vi "CMD_SERIALPARSE.vi"(6 "Gantry in":refnum<class "Gantry.lvclass">, 7 "Console Log in":refnum<class "Console Log.lvclass">, 8 "error in (no error)":errorcluster, 10 "Arguments":string[](array[string]), 11 "gScript Interpreter in":refnum<class "gScript Interpreter.lvclass">) -> (0 "error out":errorcluster, 3 "gScript Interpreter out":refnum<class "gScript Interpreter.lvclass">, 4 "Gantry out":refnum<class "Gantry.lvclass">, 5 "Console Log out":refnum<class "Console Log.lvclass">)   [LabVIEW 2024, in "gScript Interpreter.lvclass"]
uses:
  gScript Interpreter.lvclass
  Shared Components/Gantry Class/Gantry.lvclass
  Application Utilities/Console Log/Console Log.lvclass
  Type Definitions/Memory Cell.ctl
  Type Definitions/Memory Cell Type Enum.ctl
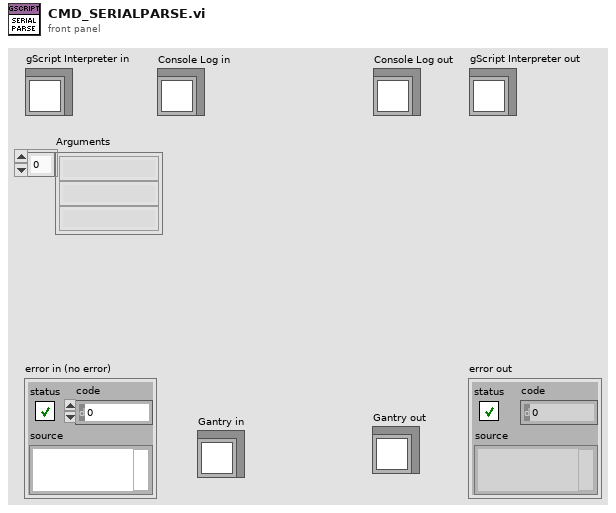
[diagram p1: front panel]
types:
  T1 = typedef "Memory Cell.ctl" = cluster{"type":T2, "x":dbl, "y":dbl, "z":dbl, "w":dbl}
  T2 = typedef "Memory Cell Type Enum.ctl" = enum16{"integer", "float", "vector", "rotation"}
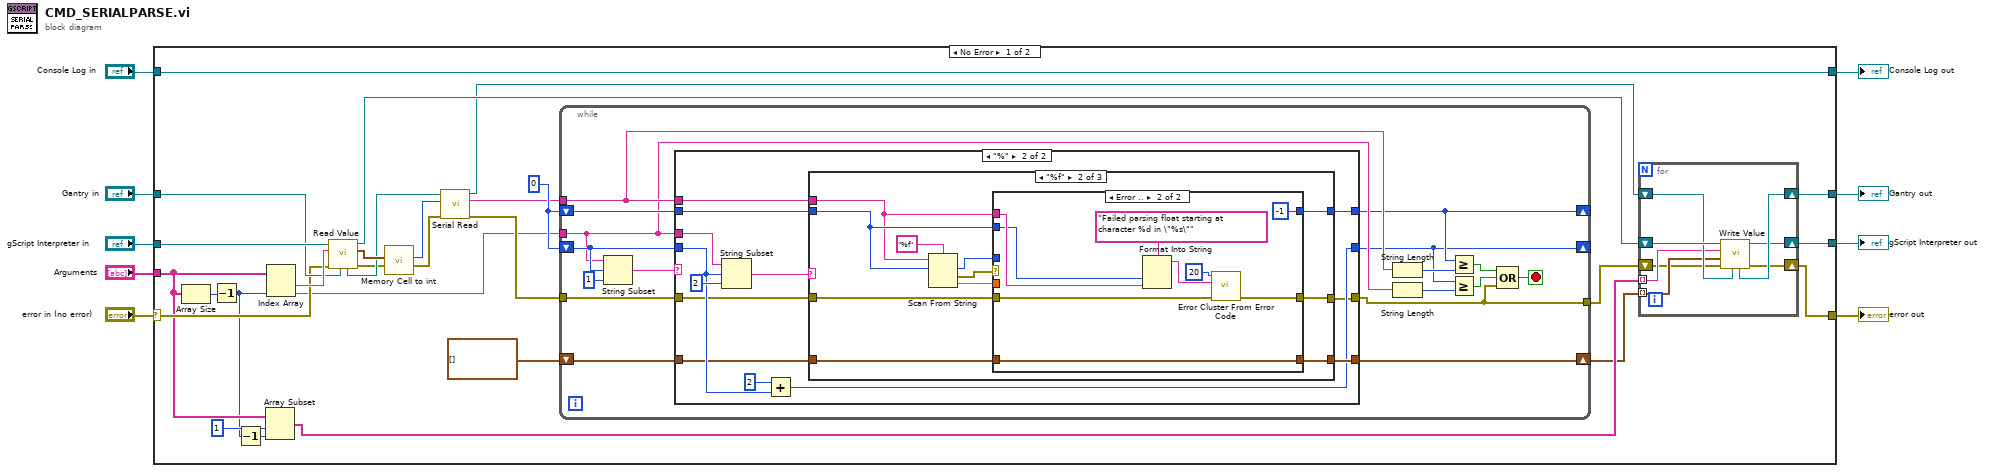
[diagram p0: block diagram]
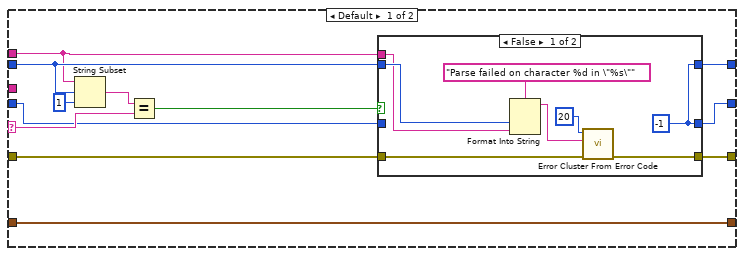
[diagram p2: hidden frame]
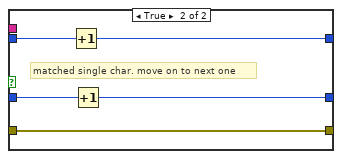
[diagram p3: hidden frame]
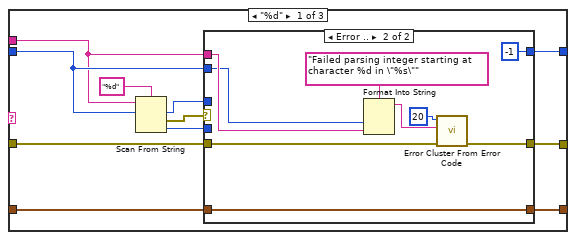
[diagram p4: hidden frame]
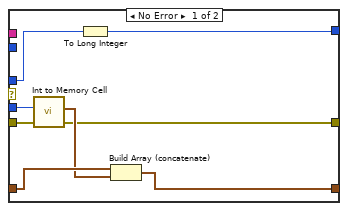
[diagram p5: hidden frame]
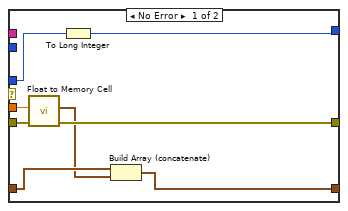
[diagram p6: hidden frame]
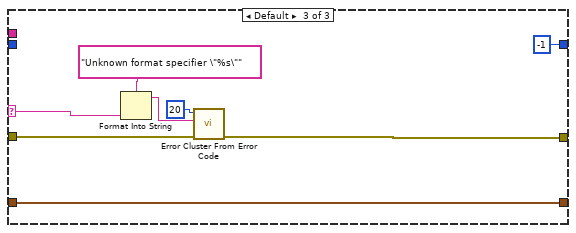
[diagram p7: hidden frame]
diagram:
  n1 = case shown="No Error" "error in (no error)" {
    selector: "error in (no error)" -> [w32 w165]
    tunnel: [w10 w165] -> w8
    tunnel: "gScript Interpreter in" -> [w34 w162]
    tunnel: "Arguments" -> [w26 _]
    tunnel: "Gantry in" -> [w33 w164]
    tunnel: [w11 w164] -> w4
    tunnel: "Console Log in" -> [w28 w163]
    tunnel: [w28 w163] -> w2
    tunnel: [w13 w162] -> w1
    frame No Error {
      w21 = 0
      n2 = Array Size(array=w26) -> (size(s)=w27:i32)
      n3 = Decrement(x=w27) -> (x-1=w24:i32)
      n4 = Decrement(x=w24) -> (x-1=w23:i32)
      n5 = Array Subset(array=w26, index=1, length=w23) -> (w17:string[])
      n6 = Index Array(array=w26, index #2=w24) -> (element #1=w36:string, element #2=w18:string)  [unwired: 1 in]
      n7 = call-dynamic "Read Value.vi"("Gantry in"=w33, "error in (no error)"=w32, "String in"=w36, "gScript Interpreter in"=w34) -> ("error out"=w30:errorcluster, "Memory Cell"=w35:T1, "gScript Interpreter out"=w14:refnum<class "gScript Interpreter.lvclass">, "Gantry out"=w31:refnum<class "Gantry.lvclass">)  [unwired: 4 in]
      n8 = call "Memory Cell to int.vi"("Memory Cell"=w35) -> ("Int out"=w29:i32)  [unwired: 10 in]
      n9 = call "Serial Read.vi"("error in (no error)"=w30, "Connection ID"=w29, "Gantry in"=w31) -> ("error out"=w22:errorcluster, "read buffer"=w19:string, "Gantry out"=w12:refnum<class "Gantry.lvclass">)  [unwired: 6 in]
      n10 = while {
        tunnel: w19 -> [w55]
        tunnel: w18 -> [w54]
        tunnel: w22 -> [w57]
        shift-right: [w53] -> _
        shift-left: w21 -> [w59]
        shift-right: [w50] -> _
        shift-left: w21 -> [w58]
        shift-right: [w45] -> w16
        shift-left: T1[] [] -> [w56]
        tunnel: [w46] -> w15
        stop <- w47 stop-if-true
        n11 = String Subset(string=w54, offset (0)=w58, length (rest)=1 ("length (rest)")) -> (substring=w60:string)
        n12 = case shown="\"%\"" w60 {
          selector: w60 -> [w71 _]
          tunnel: w54 -> [_ w98]
          tunnel: w55 -> [w63 w96]
          tunnel: w59 -> [w70 w95]
          tunnel: w58 -> [w68 w94]
          tunnel: [w69 w88] -> w53
          tunnel: [w66 w89] -> w50
          tunnel: w57 -> [w65 w91]
          tunnel: [w64 w87] -> w46
          tunnel: w56 -> [w62 w92]
          tunnel: [w62 w90] -> w45
          frame Default {
            n13 = String Subset(string=w63, offset (0)=w70, length (rest)=1 ("length (rest)")) -> (substring=w72:string)
            n14 = Equal?(x=w72, y=w71) -> (x = y?=w67:bool)
            n15 = case shown="False" w67 {
              tunnel: w70 -> [w77 w86]
              tunnel: [w74 w85] -> w69
              tunnel: w68 -> [_ w84]
              tunnel: [w74 w83] -> w66
              tunnel: w65 -> [w81 w82]
              tunnel: [w80 w82] -> w64
              tunnel: w63 -> [w76 _]
              frame False {
                w74 = -1
                n16 = Format Into String(format string="Parse failed on character %d in \"%s\"", w77, w76) -> (resulting string=w75:string)  [unwired: 2 in, 1 out]
                n17 = call <vilib>:"Error Cluster From Error Code.vi"("error in (no error)"=w81, "error message (\"\")"=w75, "error code (0)"=20) -> ("error out"=w80:errorcluster)  [unwired: 6 in]
              }
              frame True {
                # "matched single char. move on to next one"
                n18 = Increment(x=w86) -> (x+1=w85:i32)
                n19 = Increment(x=w84) -> (x+1=w83:i32)
              }
            }
          }
          frame "%" {
            n20 = String Subset(string=w98, offset (0)=w94, length (rest)=2 ("length (rest)")) -> (substring=w97:string)
            n21 = Add(x=2, y=w94) -> (x+y=w89:i32)
            n22 = case shown="\"%f\"" w97 {
              selector: w97 -> [_ _ w157]
              tunnel: w96 -> [w106 w133 _]
              tunnel: w95 -> [w107 w134 _]
              tunnel: w92 -> [w105 w132 w155]
              tunnel: w91 -> [w108 w135 w159]
              tunnel: [w104 w131 w155] -> w90
              tunnel: [w101 w128 -1] -> w88
              tunnel: [w100 w127 w156] -> w87
              frame "%d" {
                n23 = Scan From String(format string="%d", input string=w106, initial scan location=w107) -> (offset past scan=w103:u32, error out=w109:errorcluster, output 1=w102:i32)  [unwired: 2 in, 1 out]
                n24 = case shown="Error .." w109 {
                  tunnel: w108 -> [w114 w123]
                  tunnel: w107 -> [_ w121]
                  tunnel: w106 -> [_ w122]
                  tunnel: [w114 w120] -> w100
                  tunnel: w105 -> [w116 w119]
                  tunnel: [w113 w119] -> w104
                  tunnel: w103 -> [w112 _]
                  tunnel: w102 -> [w117 _]
                  tunnel: [w111 -1] -> w101
                  frame No Error {
                    n25 = call "Int to Memory Cell.vi"("Numeric"=w117) -> ("Memory Cell"=w115:T1)  [unwired: 10 in]
                    n26 = To Long Integer(number=w112) -> (32bit integer=w111:i32)
                    n27 = Build Array (concatenate)(w116, w115) -> (w113:T1[])
                  }
                  frame Error {
                    n28 = Format Into String(format string="Failed parsing integer starting at character %d in \"%s\"", w121, w122) -> (resulting string=w124:string)  [unwired: 2 in, 1 out]
                    n29 = call <vilib>:"Error Cluster From Error Code.vi"("error in (no error)"=w123, "error message (\"\")"=w124, "error code (0)"=20) -> ("error out"=w120:errorcluster)  [unwired: 6 in]
                  }
                }
              }
              frame "%f" {
                n30 = Scan From String(format string="%f", input string=w133, initial scan location=w134) -> (offset past scan=w130:u32, error out=w136:errorcluster, output 1=w129:dbl)  [unwired: 2 in, 1 out]
                n31 = case shown="Error .." w136 {
                  tunnel: w135 -> [w143 w150]
                  tunnel: w134 -> [_ w148]
                  tunnel: w133 -> [_ w149]
                  tunnel: [w143 w147] -> w127
                  tunnel: w132 -> [w144 w146]
                  tunnel: [w142 w146] -> w131
                  tunnel: w130 -> [w139 _]
                  tunnel: w129 -> [w141 _]
                  tunnel: [w138 -1] -> w128
                  frame No Error {
                    n32 = call "Float to Memory Cell.vi"("Float in"=w141) -> ("Memory Cell"=w140:T1)  [unwired: 10 in]
                    n33 = To Long Integer(number=w139) -> (32bit integer=w138:i32)
                    n34 = Build Array (concatenate)(w144, w140) -> (w142:T1[])
                  }
                  frame Error {
                    n35 = Format Into String(format string="Failed parsing float starting at character %d in \"%s\"", w148, w149) -> (resulting string=w151:string)  [unwired: 2 in, 1 out]
                    n36 = call <vilib>:"Error Cluster From Error Code.vi"("error in (no error)"=w150, "error message (\"\")"=w151, "error code (0)"=20) -> ("error out"=w147:errorcluster)  [unwired: 6 in]
                  }
                }
              }
              frame Default {
                n37 = Format Into String(format string="Unknown format specifier \"%s\"", w157) -> (resulting string=w160:string)  [unwired: 2 in, 1 out]
                n38 = call <vilib>:"Error Cluster From Error Code.vi"("error in (no error)"=w159, "error message (\"\")"=w160, "error code (0)"=20) -> ("error out"=w156:errorcluster)  [unwired: 6 in]
              }
            }
          }
        }
        n39 = String Length(string=w55) -> (length=w52:i32)
        n40 = String Length(string=w54) -> (length=w51:i32)
        n41 = Greater Or Equal?(x=w53, y=w52) -> (x >= y?=w49:bool)
        n42 = Greater Or Equal?(x=w50, y=w51) -> (x >= y?=w48:bool)
        n43 = Compound Arithmetic op=OR(w49, w48, w46) -> (w47:bool)
      }
      n44 = for {
        tunnel: w17 -> [w40] mode=indexing
        tunnel: w16 -> [w39] mode=indexing
        shift-right: [w41] -> w13
        shift-left: w14 -> [w44]
        shift-right: [w42] -> w11
        shift-left: w12 -> [w43]
        shift-right: [w37] -> w10
        shift-left: w15 -> [w38]
        n45 = call-dynamic "Write Value.vi"("Gantry in"=w43, "error in (no error)"=w38, "Value"=w39, "Address"=w40, "gScript Interpreter in"=w44) -> ("error out"=w37:errorcluster, "gScript Interpreter out"=w41:refnum<class "gScript Interpreter.lvclass">, "Gantry out"=w42:refnum<class "Gantry.lvclass">)  [unwired: 4 in]
      }
    }
    frame Error {
    }
  }
  "error out" <- w8
  "gScript Interpreter out" <- w1
  "Gantry out" <- w4
  "Console Log out" <- w2
